vi "punto #1.vi"() -> ()   [LabVIEW 2019]
panel:
  out "vaciado":bool
  out "Llenado":bool
  in  "RATA(5°C/seg)":dbl(knob) scale=0.0..10.0
  in  "SELECTOR":bool
  out "Sensor de temperatura":dbl(slide) scale=0.0..100.0
  # "Incrementar"
  # "Decrementar"
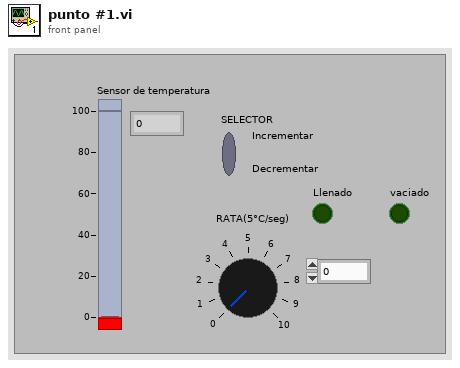
[diagram p1: front panel]
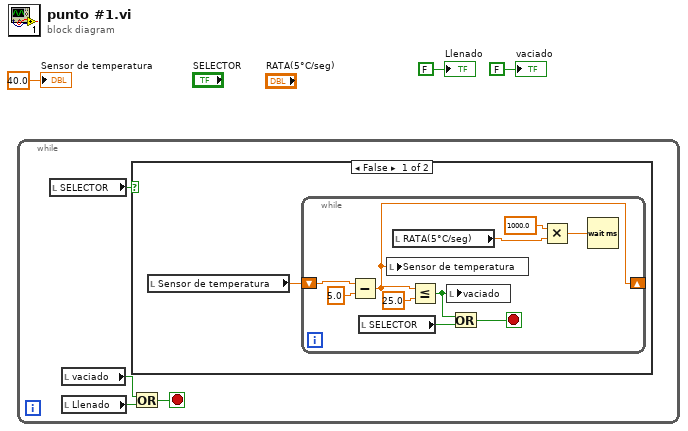
[diagram p0: block diagram]
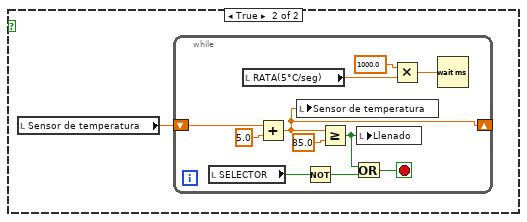
[diagram p2: hidden frame]
diagram:
  n1 = while {
    stop <- w6 stop-if-true
    n2 = local read "SELECTOR"() -> (w7:bool)
    n3 = local read "vaciado"() -> (w5:bool)
    n4 = local read "Llenado"() -> (w4:bool)
    n5 = case shown="False" w7 {
      frame False {
        n6 = local read "Sensor de temperatura"() -> (w8:dbl)
        n7 = while {
          shift-right: [w17] -> _
          shift-left: w8 -> [w18]
          stop <- w9 stop-if-true
          n8 = Subtract(x=w18, y=5.0) -> (x-y=w17:dbl)
          n9 = local read "SELECTOR"() -> (w11:bool)
          n10 = local write "Sensor de temperatura"(w17) -> ()
          n11 = local read "RATA(5°C/seg)"() -> (w13:dbl)
          n12 = Less Or Equal?(x=w17, y=25.0) -> (x <= y?=w10:bool)
          n13 = local write "vaciado"(w10) -> ()
          n14 = Or(x=w10, y=w11) -> (x .or. y?=w9:bool)
          n15 = Multiply(x=1000.0, y=w13) -> (x*y=w14:dbl)
          n16 = Wait (ms)(milliseconds to wait=w14) -> ()  [unwired: 1 out]
        }
      }
      frame True {
        n17 = local read "Sensor de temperatura"() -> (w19:dbl)
        n18 = while {
          shift-right: [w25] -> _
          shift-left: w19 -> [w30]
          stop <- w23 stop-if-true
          n19 = local read "SELECTOR"() -> (w21:bool)
          n20 = local read "RATA(5°C/seg)"() -> (w27:dbl)
          n21 = Add(x=w30, y=5.0) -> (x+y=w25:dbl)
          n22 = local write "Sensor de temperatura"(w25) -> ()
          n23 = Not(x=w21) -> (.not. x?=w22:bool)
          n24 = Greater Or Equal?(x=w25, y=85.0) -> (x >= y?=w20:bool)
          n25 = Or(x=w20, y=w22) -> (x .or. y?=w23:bool)
          n26 = local write "Llenado"(w20) -> ()
          n27 = Multiply(x=1000.0, y=w27) -> (x*y=w28:dbl)
          n28 = Wait (ms)(milliseconds to wait=w28) -> ()  [unwired: 1 out]
        }
      }
    }
    n29 = Or(x=w5, y=w4) -> (x .or. y?=w6:bool)
  }
  "Sensor de temperatura" <- 40.0 ("Sensor de temperatura")
  "Llenado" <- FALSE ("Llenado")
  "vaciado" <- FALSE ("vaciado")
